vi "configuration UI.vi"() -> ()   [LabVIEW 2013, in "Scan Engine editor node.lvclass"]
uses:
  Scan Engine editor node.lvclass
  <vilib>/NI/Configuration Framework/Node/NodeRef.ctl
  <vilib>/NI/Configuration Framework/Node/NISE_CEF_Node.lvclass
  <vilib>/NI/AMC/Message Queue.ctl
  <vilib>/NI/AMC/Message.ctl
  <vilib>/NI/Tools/Keyed Array/KeyedArray.ctl
  <vilib>/NI/Configuration Framework/Node/UserEventRef.ctl
  <vilib>/NI/Configuration Framework/Controls/EventCluster.ctl
  module/configuration/Scan Engine configuration.lvclass
  <vilib>/Utility/miscctls.llb/LVComboBoxStrsAndValuesArrayTypeDef.ctl
  module/configuration/Scan Engine configuration.lvclass/Scan Engine configuration.ctl
  <vilib>/NI/Configuration Framework/serializable configuration/NISE_CEF_serializable configuration.lvclass/NISE_CEF_serializable configuration.ctl
  <vilib>/NI/Configuration Framework/serializable configuration/NISE_CEF_serializable configuration.lvclass
  Scan Engine editor node.lvclass/Scan Engine editor node.ctl
  <vilib>/NI/Tag Bus/tag/tag descriptor.lvclass/tag descriptor.ctl
  <vilib>/NI/Tag Bus Module Framework/module configuration/TBM module configuration.lvclass
  module/configuration/Write discover channels.vi
  module/configuration/Read discover channels.vi
  <vilib>/NI/Configuration Framework/serializable configuration/Read UID.vi
  <vilib>/NI/Tag Bus Data Framework/Configuration Editor/Classes/Module editor node/Read Module Configuration.vi
  read actual configuration.vi
  <vilib>/NI/Module Execution Interface/Engine Configuration/engine configuration.lvclass
  <vilib>/NI/Tag Bus Data Framework/Configuration Editor/Classes/Module editor node/module editor node.lvclass
  <vilib>/NI/Tag Bus/tag/tag descriptor.lvclass
  <vilib>/NI/Configuration Framework/NISE_CEF_TreeControl.lvlib
  <vilib>/NI/Tag Bus Data Framework/Configuration Editor/Classes/Engine Parent/Engine Parent Editor Node.lvclass
  <vilib>/Utility/miscctls.llb/LVRowAndColumnUnsignedTypeDef.ctl
  <vilib>/NI/Tools/Keyed Array/Tools_KeyedArray.lvlib
  <vilib>/NI/AMC/AMC.lvlib
panel:
  in  "hidden_settings":bool
  in  "Tab Control":enum32{"Static Configuration"}(tab)
  in  "Generate Tags":bool
  in  "Discover Channels?":bool
  in  "Remove Button":bool
  in  "Add Button":bool
  in  "channels":i32(listbox)
  in  "settings":bool
  in  "Import":bool
  in  "Tag":string(combo)
  in  "scan period (uSec)":u32=10000
  in  "user event":T1
  in  "main queue":T2
  in  "node ref":T3
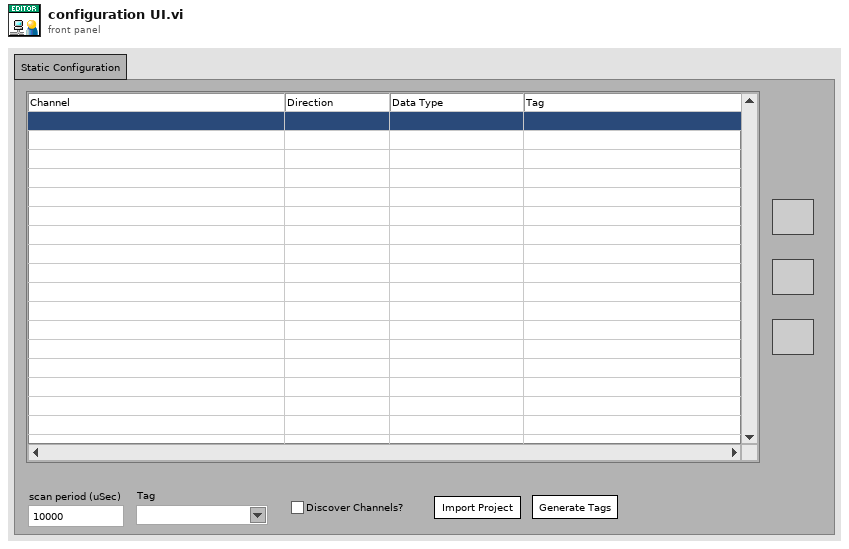
[diagram p1: front panel]
types:
  T1 = typedef "NISE_CEF_Node.lvclass/UserEventRef.ctl" = refnum<user-event>
  T2 = typedef "AMC.lvlib/Message Queue.ctl" = refnum<queue>
  T3 = typedef "NISE_CEF_Node.lvclass/NodeRef.ctl" = refnum<data-value>
  T4 = enum32{"invalid app kind", "Development System", "Run Time System", "Student Edition", "Embedded LabVIEW", "Evaluation", "Custom"}
  T5 = typedef "LVComboBoxStrsAndValuesArrayTypeDef.ctl" = cluster{"String":string, "Value":string}[]
  T6 = typedef "NISE_CEF_TreeControl.lvlib/EventCluster.ctl" = cluster{"command":string, "data":string}
  T7 = typedef "LVRowAndColumnUnsignedTypeDef.ctl" = cluster{"Row":u32, "Column":u32}
  T8 = typedef "Scan Engine editor node.lvclass/table line.ctl" = cluster{"tag":string, "channel":refnum<class "TBM channel.lvclass">}
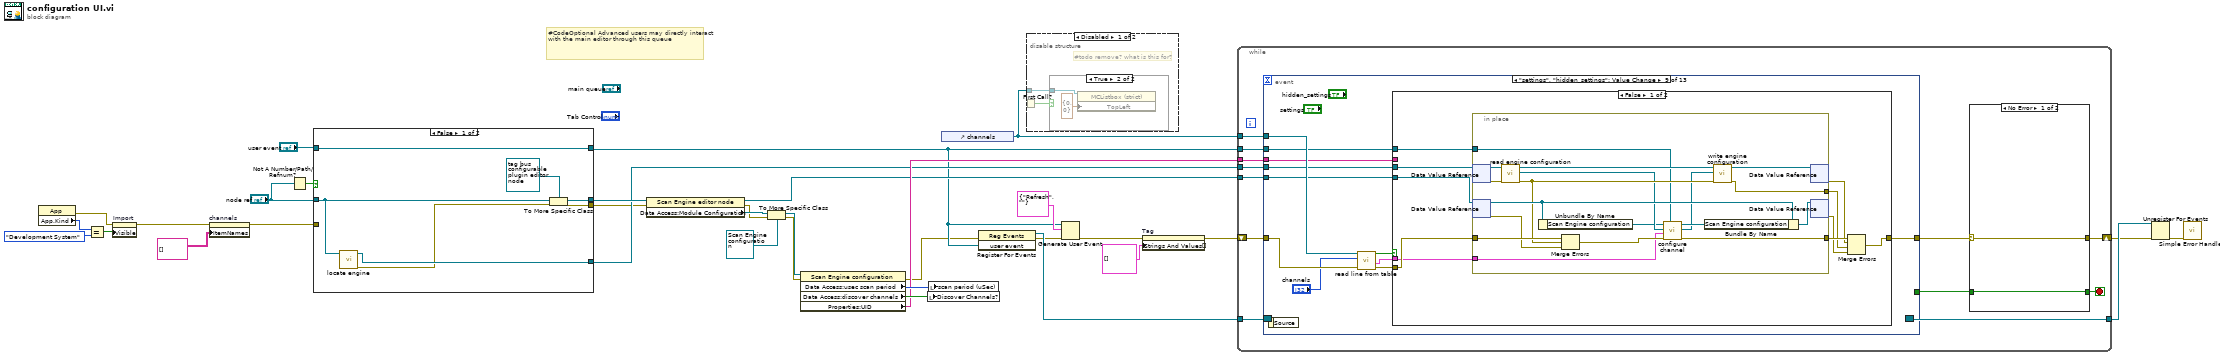
[diagram p0: block diagram]
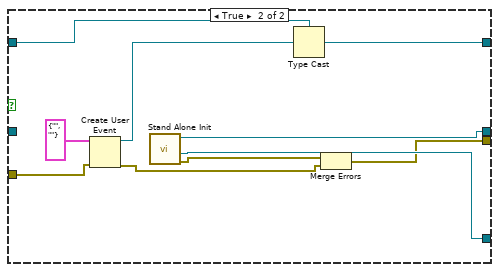
[diagram p4: hidden frame]
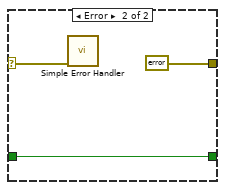
[diagram p5: hidden frame]
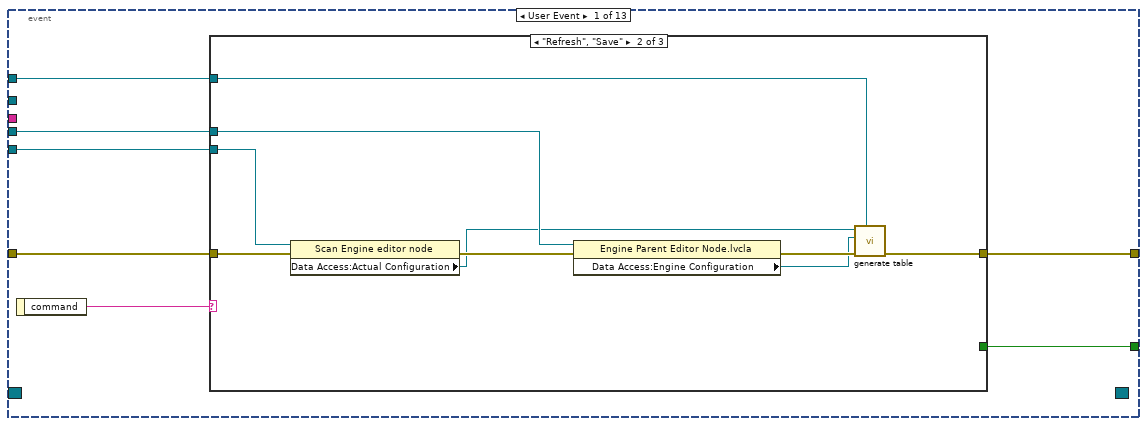
[diagram p6: hidden frame]
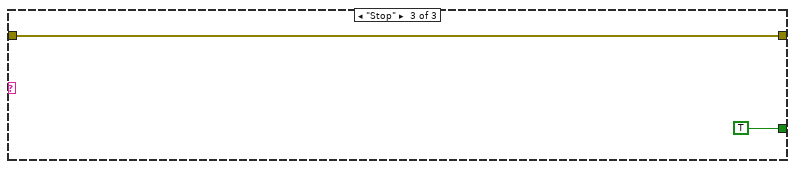
[diagram p8: hidden frame]
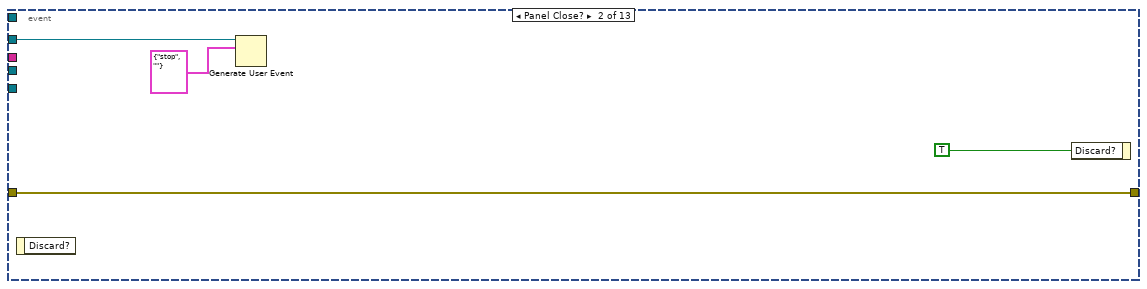
[diagram p9: hidden frame]
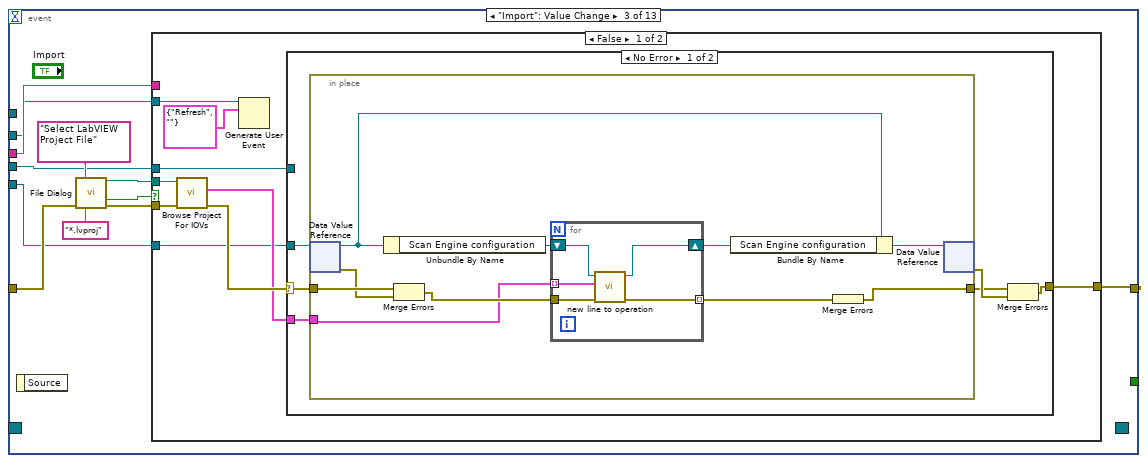
[diagram p10: hidden frame]
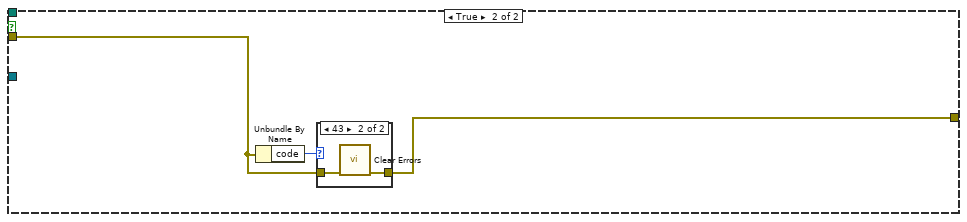
[diagram p12: hidden frame]
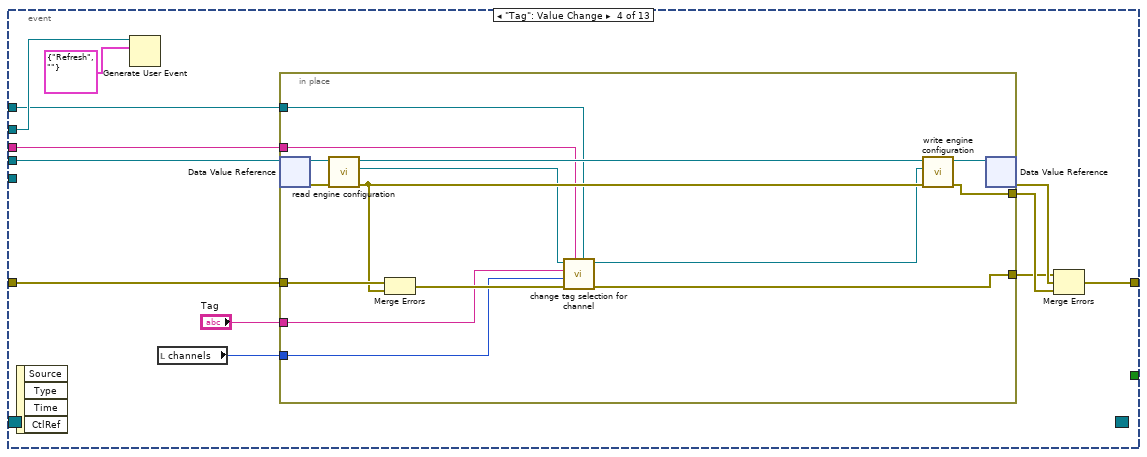
[diagram p14: hidden frame]
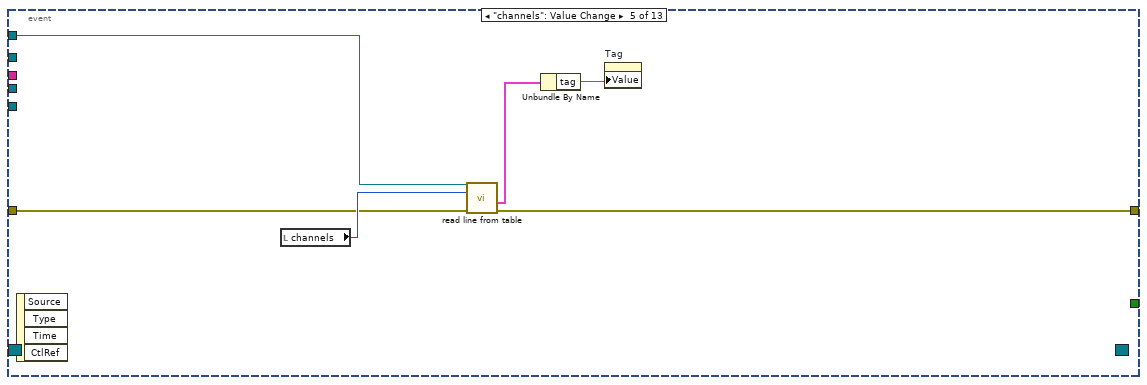
[diagram p15: hidden frame]
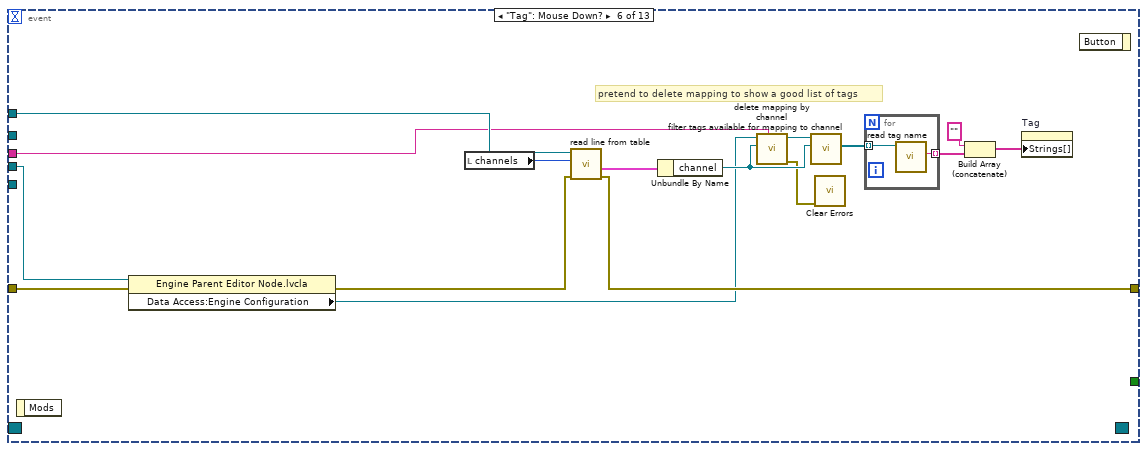
[diagram p16: hidden frame]
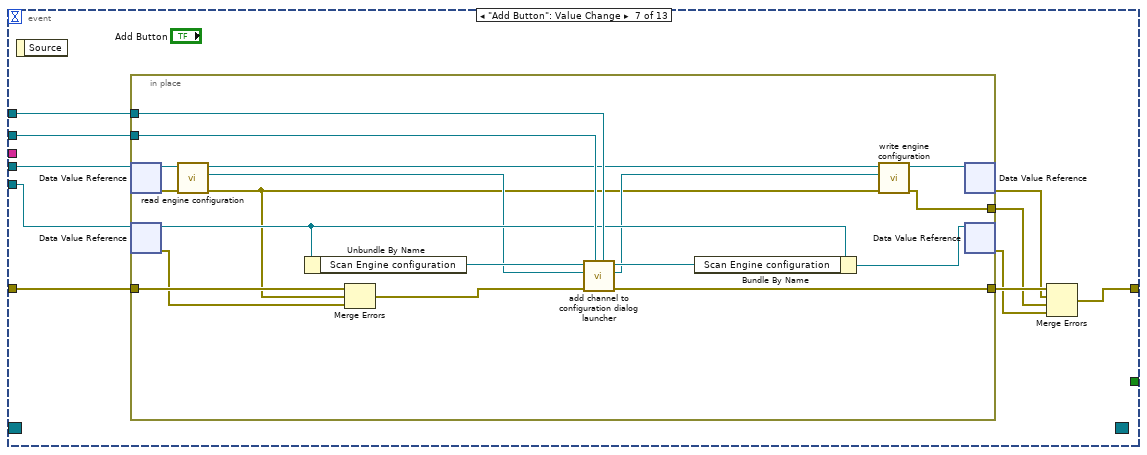
[diagram p17: hidden frame]
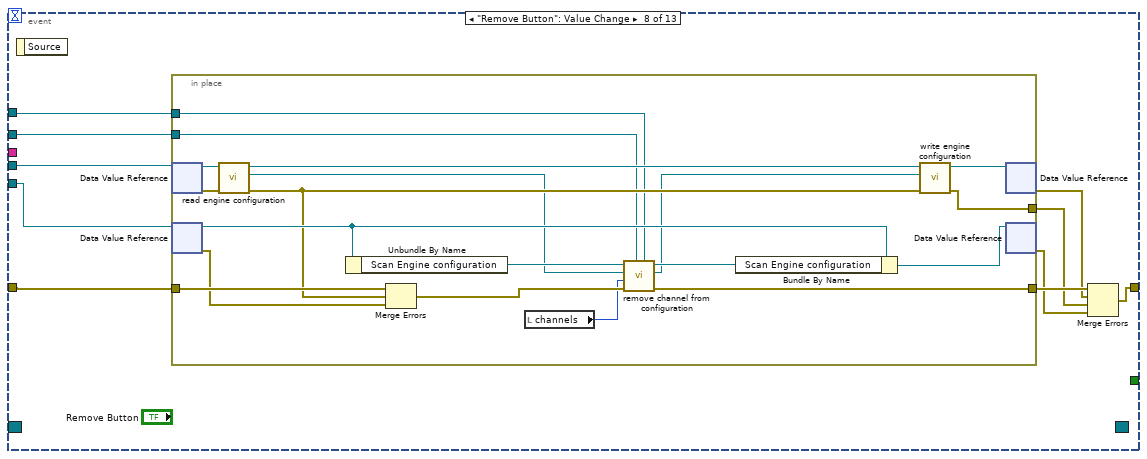
[diagram p18: hidden frame]
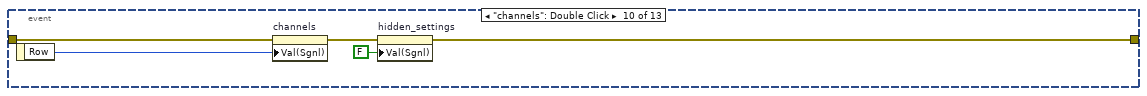
[diagram p20: hidden frame]
diagram:
  # "#CodeOptional Advanced users may directly interact with the main editor through this queue"
  n1 = property class="App"() -> (error out=w2:errorcluster, "App.Kind"=w5:T4)  [unwired: 2 in, 1 out]
  n2 = Equal?(x=w5, y=T4."Development System") -> (x = y?=w3:bool)
  n3 = property on="Import" class="Bool"(error in=w2, "Visible"=w3) -> (error out=w1:errorcluster)  [unwired: 1 in, 1 out]
  n4 = property on="channels" class="MCListbox (strict)"(error in=w1, "ItemNames"=string[][] [] ("Item Names")) -> (error out=w19:errorcluster)  [unwired: 1 in, 1 out]
  n5 = Not A Number/Path/Refnum?(number/path/refnum="node ref") -> (NaN/Path/Refnum?=w28:bool)
  n6 = case shown="False" w28 {
    tunnel: "user event" -> [w41 w42]
    tunnel: [w41 w43] -> w13
    tunnel: "node ref" -> [w39 _]
    tunnel: [w38 w51] -> w21
    tunnel: [w37 w45] -> w10
    tunnel: [w36 w49] -> w15
    tunnel: w19 -> [_ w46]
    frame False {
      n7 = call <vilib>:"locate engine.vi"("component"=w39) -> ("error out"=w35:errorcluster, "engine"=w36:refnum<data-value>)  [unwired: 9 in]
      n8 = To More Specific Class(target class=refnum<data-value> refnum ("data value reference"), reference=w39, error in=w35) -> (specific class reference=w38:refnum<data-value>, error out=w37:errorcluster)
    }
    frame True {
      n9 = Create User Event(user event datatype=T6 {"command"="", "data"=""} ("event data"), error in=w46) -> (user event=w47:refnum<user-event>, error out=w44:errorcluster)
      n10 = call "Stand Alone Init.vi"() -> ("error out"=w50:errorcluster, "Engine Parent Editor Node"=w49:refnum<data-value>, "Scan Engine Editor Node"=w51:refnum<data-value>)  [unwired: 9 in]
      n11 = Type Cast(type=w42, x=w47) -> (*(type *) &x=w43:T1)
      n12 = Merge Errors(w50, w44) -> (w45:errorcluster)
    }
  }
  n13 = property class="Scan Engine editor node"(reference=w21, error in=w10) -> (reference out=w16:refnum<data-value>, error out=w9:errorcluster, "Data Access:Module Configuration"=w24:refnum<class "TBM module configuration.lvclass">)
  n14 = To More Specific Class(target class=refnum<class "Scan Engine configuration.lvclass"> refnum ("Scan Engine configuration"), reference=w24, error in=w9) -> (specific class reference=w23:refnum<class "Scan Engine configuration.lvclass">, error out=w8:errorcluster)
  n15 = property class="Scan Engine configuration"(reference=w23, error in=w8) -> (error out=w7:errorcluster, "Data Access:usec scan period"=w30:u32, "Data Access:discover channels"=w29:bool, "Properties:UID"=w20:string)  [unwired: 1 out]
  n16 = local write "Discover Channels?"(w29) -> ()
  n17 = local write "scan period (uSec)"(w30) -> ()
  n18 = control-ref of="channels"() -> (w22:refnum<vi>)
  n19 = register-events(error in=w7, w13) -> (reference out=w34:refnum<event-registration>, error out=w12:errorcluster)  [unwired: 1 in]
  n20 = disable-structure shown="Disabled" {
    disable-tunnel: w22 -> [w52 _]
    frame Disabled {
      # "#todo remove? what is this for?"
      n21 = First Call?() -> (First Call?: T/F=w53:bool)
      n22 = case shown="True" w53 {
        tunnel: w52 -> [_ w54]
        frame False {
        }
        frame True {
          n23 = property class="MCListbox (strict)"(reference=w54, "TopLeft"=T7 {"Row"=0, "Column"=0} ("Top Left Visible Cell")) -> ()  [unwired: 1 in, 2 out]
        }
      }
    }
    frame Enabled {
    }
  }
  n24 = Generate User Event(user event=w13, event data cluster=T6 {"command"="Refresh", "data"=""} ("event data"), error in=w12) -> (error out=w11:errorcluster)  [unwired: 1 in, 1 out]
  n25 = property on="Tag" class="CmbBox"(error in=w11, "Strings And Values[]"=T5 [] ("Strings And Values []")) -> (error out=w31:errorcluster)  [unwired: 1 in, 1 out]
  n26 = while {
    tunnel: w34 -> [w67]
    tunnel: [w66] -> w33
    shift-right: [w62] -> w32
    shift-left: w31 -> [w65]
    tunnel: w22 -> [w57]
    tunnel: w20 -> [w61]
    tunnel: w16 -> [w59]
    tunnel: w15 -> [w58]
    tunnel: w13 -> [w56]
    stop <- w64 stop-if-true
    n27 = event shown="[8] \"settings\", \"hidden_settings\": Value Change" {
      selector: w67 -> [_ _ _ _ _ _ _ _ _ _ _ _ _]
      dyn-events: [_ _ _ _ _ _ _ _ _ _ _ _ _] -> w66
      timeout: _ -> [_ _ _ _ _ _ _ _ _ _ _ _ _]
      tunnel: [w78 _ _ _ _ _ _ _ _ _ _ _ _] -> w63
      tunnel: [w76 w95 w102 w151 w174 w185 w198 w228 w259 w294 w301 w316 w334] -> w60
      tunnel: w65 -> [w77 w95 w106 w150 w175 w184 w203 w227 w262 w296 w299 w314 w339]
      tunnel: w57 -> [w73 _ _ w148 w173 w189 w201 w223 w258 _ _ _ _]
      tunnel: w61 -> [_ _ w99 w149 _ w181 _ _ w257 _ _ _ w337]
      tunnel: w59 -> [w75 _ w96 _ _ _ w199 w226 w252 _ w300 w315 w332]
      tunnel: w58 -> [w74 _ w97 w144 _ w178 w200 w225 w253 _ _ _ w329]
      tunnel: w56 -> [_ w93 w98 w154 _ _ w202 w224 w255 _ _ _ w335]
      event User Event {
        n28 = event-data() -> ("command"=w79:string)  [unwired: 1 in]
        n29 = case shown="\"Refresh\", \"Save\"" w79 {
          tunnel: [_ _ TRUE] -> w78
          tunnel: w77 -> [w80 w88 w90]
          tunnel: [w80 w87 w90] -> w76
          tunnel: w75 -> [_ w84 _]
          tunnel: w74 -> [_ w83 _]
          tunnel: w73 -> [_ w89 _]
          frame Default {
          }
          frame "Refresh", "Save" {
            n30 = property class="Scan Engine editor node"(reference=w84, error in=w88) -> (error out=w86:errorcluster, "Data Access:Actual Configuration"=w81:refnum<class "Scan Engine configuration.lvclass">)  [unwired: 1 out]
            n31 = property class="Engine Parent Editor Node.lvcla"(reference=w83, error in=w86) -> (error out=w85:errorcluster, "Data Access:Engine Configuration"=w82:refnum<class "engine configuration.lvclass">)  [unwired: 1 out]
            n32 = call "generate table.vi"("table"=w89, "error in"=w85, "engine configuration in"=w82, "Scan Engine configuration"=w81) -> ("error out"=w87:errorcluster)  [unwired: 7 in]
          }
          frame "Stop" {
          }
        }
      }
      event Panel Close? {
        n33 = event-data() -> ()  [unwired: 1 in, 1 out]
        n34 = Generate User Event(user event=w93, event data cluster=T6 {"command"="stop", "data"=""} ("event data")) -> ()  [unwired: 2 in, 2 out]
        n35 = event-data("Discard?"=TRUE) -> ()  [unwired: 1 in, 1 out]
      }
      event "Import": Value Change {
        n36 = event-data() -> ()  [unwired: 1 in, 1 out]
        n37 = call "File Dialog"("prompt"="Select LabVIEW Project File", "error in"=w106, "pattern (all files)"="*.lvproj") -> ("selected path"=w101:path, "cancelled"=w104:bool, "error out"=w103:errorcluster)  [unwired: 9 in, 1 out]
        n38 = case shown="False" w104 {
          tunnel: w103 -> [w114 w139]
          tunnel: [w111 w138] -> w102
          tunnel: w101 -> [w115 _]
          tunnel: w99 -> [_ _]
          tunnel: w98 -> [w112 _]
          tunnel: w97 -> [w108 _]
          tunnel: w96 -> [w107 _]
          frame False {
            n39 = call "Browse Project For IOVs.vi"("error in"=w114, "Path"=w115) -> ("error out"=w110:errorcluster, "Tags"=w109:T8[])  [unwired: 8 in]
            n40 = Generate User Event(user event=w112, event data cluster=T6 {"command"="Refresh", "data"=""} ("event data")) -> ()  [unwired: 2 in, 2 out]
            n41 = case shown="No Error" w110 {
              selector: w110 -> [w119 w137]
              tunnel: [w120 w137] -> w111
              tunnel: w109 -> [w118 _]
              tunnel: w108 -> [_ _]
              tunnel: w107 -> [w117 _]
              frame No Error {
                n42 = in-place {
                  in-place-border: w119 -> [w131]
                  in-place-border: w118 -> [w124]
                  in-place-border: [w122] -> w116
                  n43 = in-place-dvr #1(w117) -> (w129:refnum<class "Scan Engine editor node.lvclass">, w130:errorcluster)
                  n44 = Unbundle By Name(w129) -> ("Scan Engine configuration"=w127:refnum<class "Scan Engine configuration.lvclass">)
                  n45 = Merge Errors(w131, w130) -> (w125:errorcluster)
                  n46 = for {
                    shift-right: [w134] -> w126
                    shift-left: w127 -> [w135]
                    tunnel: w125 -> [w133]
                    tunnel: w124 -> [w132] mode=indexing
                    tunnel: [w136] -> w123 mode=indexing
                    n47 = call "new line to operation.vi"("error in"=w133, "new line item"=w132, "Actual Configuration"=w135) -> ("error out"=w136:errorcluster, "Scan Engine configuration out"=w134:refnum<class "Scan Engine configuration.lvclass">)  [unwired: 4 in, 3 out]
                  }
                  n48 = Bundle By Name(cluster=w129, "Scan Engine configuration"=w126) -> (w128:refnum<class "Scan Engine editor node.lvclass">)
                  n49 = Merge Errors(w123) -> (w122:errorcluster)
                  n50 = in-place-dvr #1(w128) -> (w121:errorcluster)  [unwired: 1 out]
                }
                n51 = Merge Errors(w116, w121) -> (w120:errorcluster)
              }
              frame Error {
              }
            }
          }
          frame True {
            n52 = Unbundle By Name(w139) -> ("code"=w140:i32)
            n53 = case shown="43" w140 {
              tunnel: w139 -> [w141 w143]
              tunnel: [w141 w142] -> w138
              frame Default {
              }
              frame 43 {
                n54 = call <vilib>:"Clear Errors.vi"("error in (no error)"=w143) -> ("error out"=w142:errorcluster)  [unwired: 6 in]
              }
            }
          }
        }
      }
      event "Tag": Value Change {
        n55 = event-data() -> ()  [unwired: 1 in, 4 out]
        n56 = Generate User Event(user event=w154, event data cluster=T6 {"command"="Refresh", "data"=""} ("event data")) -> ()  [unwired: 2 in, 2 out]
        n57 = local read "channels"() -> (w145:i32)
        n58 = in-place {
          in-place-border: w149 -> [w158]
          in-place-border: w150 -> [w170]
          in-place-border: [w164] -> w153
          in-place-border: w148 -> [w162]
          in-place-border: [w161] -> w147
          in-place-border: "Tag" -> [w157]
          in-place-border: w145 -> [w156]
          n59 = in-place-dvr #2(w144) -> (w169:refnum<class "Engine Parent Editor Node.lvclass">, w168:errorcluster)
          n60 = call <vilib>:"read engine configuration.vi"("error in"=w168, "Engine Parent Editor Node in"=w169) -> ("error out"=w165:errorcluster, "engine configuration"=w159:refnum<class "engine configuration.lvclass">, "Engine Parent Editor Node out"=w167:refnum<class "Engine Parent Editor Node.lvclass">)  [unwired: 7 in]
          n61 = Merge Errors(w170, w165) -> (w163:errorcluster)
          n62 = call "change tag selection for channel.vi"("channels table"=w162, "instance identifier"=w158, "error in"=w163, "channels"=w156, "Tag"=w157, "engine configuration in"=w159) -> ("error out"=w161:errorcluster, "engine configuration out"=w160:refnum<class "engine configuration.lvclass">)  [unwired: 4 in]
          n63 = call <vilib>:"write engine configuration.vi"("error in"=w165, "engine configuration"=w160, "Engine Parent Editor Node in"=w167) -> ("error out"=w164:errorcluster, "Engine Parent Editor Node out"=w166:refnum<class "Engine Parent Editor Node.lvclass">)  [unwired: 7 in]
          n64 = in-place-dvr #2(w166) -> (w152:errorcluster)  [unwired: 1 out]
        }
        n65 = Merge Errors(w147, w152, w153) -> (w151:errorcluster)
      }
      event "channels": Value Change {
        n66 = event-data() -> ()  [unwired: 1 in, 4 out]
        n67 = local read "channels"() -> (w176:i32)
        n68 = call "read line from table.vi"("error in"=w175, "line number"=w176, "operations table"=w173) -> ("error out"=w174:errorcluster, "line"=w172:T8)  [unwired: 5 in, 2 out]
        n69 = Unbundle By Name(w172) -> ("tag"=w171:string)
        n70 = property on="Tag" class="CmbBox"("Value"=w171) -> ()  [unwired: 2 in, 2 out]
      }
      event "Tag": Mouse Down? {
        # "pretend to delete mapping to show a good list of tags"
        n71 = event-data() -> ()  [unwired: 1 in, 1 out]
        n72 = property class="Engine Parent Editor Node.lvcla"(reference=w178, error in=w184) -> (error out=w179:errorcluster, "Data Access:Engine Configuration"=w177:refnum<class "engine configuration.lvclass">)  [unwired: 1 out]
        n73 = local read "channels"() -> (w188:i32)
        n74 = call "read line from table.vi"("error in"=w179, "line number"=w188, "operations table"=w189) -> ("error out"=w185:errorcluster, "line"=w187:T8)  [unwired: 5 in, 2 out]
        n75 = Unbundle By Name(w187) -> ("channel"=w182:refnum<class "TBM channel.lvclass">)
        n76 = call <vilib>:"delete mapping by channel.vi"("owner ID"=w181, "channel"=w182, "engine configuration in"=w177) -> ("error out"=w180:errorcluster, "engine configuration out"=w183:refnum<class "engine configuration.lvclass">)  [unwired: 7 in]
        n77 = call <vilib>:"filter tags available for mapping to channel.vi"("channel to map to"=w182, "engine configuration in"=w183) -> ("filtered tags"=w192:refnum<class "tag descriptor.lvclass">[])  [unwired: 8 in, 1 out]
        n78 = call <vilib>:"Clear Errors.vi"("error in (no error)"=w180) -> ()  [unwired: 6 in, 1 out]
        n79 = for {
          tunnel: w192 -> [w194] mode=indexing
          tunnel: [w193] -> w191 mode=indexing
          n80 = call <vilib>:"read tag name.vi"("system tag in"=w194) -> ("name"=w193:string)  [unwired: 8 in, 2 out]
        }
        n81 = Build Array (concatenate)("", w191) -> (w186:string[])
        n82 = property on="Tag" class="CmbBox"("Strings[]"=w186) -> ()  [unwired: 2 in, 2 out]
        n83 = event-data() -> ()  [unwired: 2 in, 1 out]
      }
      event "Add Button": Value Change {
        n84 = event-data() -> ()  [unwired: 1 in, 1 out]
        n85 = in-place {
          in-place-border: [w222] -> w204
          in-place-border: w203 -> [w221]
          in-place-border: w202 -> [w220]
          in-place-border: w201 -> [w219]
          in-place-border: [w210] -> w196
          n86 = in-place-dvr #3(w200) -> (w217:refnum<class "Engine Parent Editor Node.lvclass">, w216:errorcluster)
          n87 = in-place-dvr #4(w199) -> (w213:refnum<class "Scan Engine editor node.lvclass">, w215:errorcluster)
          n88 = call <vilib>:"read engine configuration.vi"("error in"=w216, "Engine Parent Editor Node in"=w217) -> ("error out"=w205:errorcluster, "engine configuration"=w207:refnum<class "engine configuration.lvclass">, "Engine Parent Editor Node out"=w208:refnum<class "Engine Parent Editor Node.lvclass">)  [unwired: 7 in]
          n89 = Unbundle By Name(w213) -> ("Scan Engine configuration"=w214:refnum<class "Scan Engine configuration.lvclass">)
          n90 = Merge Errors(w221, w205, w215) -> (w218:errorcluster)
          n91 = call "add channel to configuration dialog launcher.vi"("channels"=w219, "user event"=w220, "error in"=w218, "engine configuration.lvclass in"=w207, "Scan Engine configuration in"=w214) -> ("error out"=w222:errorcluster, "engine configuration.lvclass out"=w206:refnum<class "engine configuration.lvclass">, "Scan Engine configuration out"=w212:refnum<class "Scan Engine configuration.lvclass">)  [unwired: 4 in]
          n92 = Bundle By Name(cluster=w213, "Scan Engine configuration"=w212) -> (w211:refnum<class "Scan Engine editor node.lvclass">)
          n93 = call <vilib>:"write engine configuration.vi"("error in"=w205, "engine configuration"=w206, "Engine Parent Editor Node in"=w208) -> ("error out"=w210:errorcluster, "Engine Parent Editor Node out"=w209:refnum<class "Engine Parent Editor Node.lvclass">)  [unwired: 7 in]
          n94 = in-place-dvr #3(w209) -> (w195:errorcluster)  [unwired: 1 out]
          n95 = in-place-dvr #4(w211) -> (w197:errorcluster)  [unwired: 1 out]
        }
        n96 = Merge Errors(w204, w195, w196, w197) -> (w198:errorcluster)
      }
      event "Remove Button": Value Change {
        n97 = event-data() -> ()  [unwired: 1 in, 1 out]
        n98 = in-place {
          in-place-border: [w239] -> w232
          in-place-border: w227 -> [w251]
          in-place-border: w224 -> [w240]
          in-place-border: w223 -> [w241]
          in-place-border: [w245] -> w230
          n99 = in-place-dvr #5(w225) -> (w250:refnum<class "Engine Parent Editor Node.lvclass">, w249:errorcluster)
          n100 = in-place-dvr #6(w226) -> (w247:refnum<class "Scan Engine editor node.lvclass">, w248:errorcluster)
          n101 = call <vilib>:"read engine configuration.vi"("error in"=w249, "Engine Parent Editor Node in"=w250) -> ("error out"=w242:errorcluster, "engine configuration"=w234:refnum<class "engine configuration.lvclass">, "Engine Parent Editor Node out"=w243:refnum<class "Engine Parent Editor Node.lvclass">)  [unwired: 7 in]
          n102 = Unbundle By Name(w247) -> ("Scan Engine configuration"=w237:refnum<class "Scan Engine configuration.lvclass">)
          n103 = Merge Errors(w251, w242, w248) -> (w238:errorcluster)
          n104 = local read "channels"() -> (w233:i32)
          n105 = call "remove channel from configuration.vi"("channels"=w241, "user event"=w240, "error in"=w238, "channels value"=w233, "engine configuration in"=w234, "Scan Engine configuration in"=w237) -> ("error out"=w239:errorcluster, "engine configuration out"=w235:refnum<class "engine configuration.lvclass">, "Scan Engine configuration out"=w236:refnum<class "Scan Engine configuration.lvclass">)  [unwired: 3 in]
          n106 = Bundle By Name(cluster=w247, "Scan Engine configuration"=w236) -> (w246:refnum<class "Scan Engine editor node.lvclass">)
          n107 = call <vilib>:"write engine configuration.vi"("error in"=w242, "engine configuration"=w235, "Engine Parent Editor Node in"=w243) -> ("error out"=w245:errorcluster, "Engine Parent Editor Node out"=w244:refnum<class "Engine Parent Editor Node.lvclass">)  [unwired: 7 in]
          n108 = in-place-dvr #5(w244) -> (w229:errorcluster)  [unwired: 1 out]
          n109 = in-place-dvr #6(w246) -> (w231:errorcluster)  [unwired: 1 out]
        }
        n110 = Merge Errors(w232, w229, w230, w231) -> (w228:errorcluster)
      }
      event "settings", "hidden_settings": Value Change {
        n111 = event-data() -> ()  [unwired: 1 in, 1 out]
        n112 = call "read line from table.vi"("error in"=w262, "line number"="channels", "operations table"=w258) -> ("error out"=w261:errorcluster, "line"=w256:T8, "empty channel?"=w254:bool)  [unwired: 5 in, 1 out]
        n113 = case shown="False" w254 {
          tunnel: w261 -> [w265 w291]
          tunnel: [w268 w291] -> w259
          tunnel: w257 -> [_ _]
          tunnel: w256 -> [w264 _]
          tunnel: w255 -> [w263 _]
          tunnel: w253 -> [w267 _]
          tunnel: w252 -> [w266 _]
          frame False {
            n114 = in-place {
              in-place-border: [w279] -> w272
              in-place-border: w265 -> [w290]
              in-place-border: w263 -> [w273]
              in-place-border: [w284] -> w270
              in-place-border: w264 -> [w274]
              n115 = in-place-dvr #7(w267) -> (w289:refnum<class "Engine Parent Editor Node.lvclass">, w288:errorcluster)
              n116 = in-place-dvr #8(w266) -> (w286:refnum<class "Scan Engine editor node.lvclass">, w287:errorcluster)
              n117 = call <vilib>:"read engine configuration.vi"("error in"=w288, "Engine Parent Editor Node in"=w289) -> ("error out"=w281:errorcluster, "engine configuration"=w276:refnum<class "engine configuration.lvclass">, "Engine Parent Editor Node out"=w282:refnum<class "Engine Parent Editor Node.lvclass">)  [unwired: 7 in]
              n118 = Unbundle By Name(w286) -> ("Scan Engine configuration"=w275:refnum<class "Scan Engine configuration.lvclass">)
              n119 = Merge Errors(w290, w281, w287) -> (w280:errorcluster)
              n120 = call "configure channel.vi"("user event"=w273, "error in"=w280, "line"=w274, "engine configuration in"=w276, "Scan Engine configuration in"=w275) -> ("error out"=w279:errorcluster, "engine configuration out"=w277:refnum<class "engine configuration.lvclass">, "Scan Engine configuration out"=w278:refnum<class "Scan Engine configuration.lvclass">)  [unwired: 4 in]
              n121 = Bundle By Name(cluster=w286, "Scan Engine configuration"=w278) -> (w285:refnum<class "Scan Engine editor node.lvclass">)
              n122 = call <vilib>:"write engine configuration.vi"("error in"=w281, "engine configuration"=w277, "Engine Parent Editor Node in"=w282) -> ("error out"=w284:errorcluster, "Engine Parent Editor Node out"=w283:refnum<class "Engine Parent Editor Node.lvclass">)  [unwired: 7 in]
              n123 = in-place-dvr #7(w283) -> (w269:errorcluster)  [unwired: 1 out]
              n124 = in-place-dvr #8(w285) -> (w271:errorcluster)  [unwired: 1 out]
            }
            n125 = Merge Errors(w272, w269, w270, w271) -> (w268:errorcluster)
          }
          frame True {
          }
        }
      }
      event "channels": Double Click {
        n126 = event-data() -> ("Row"=w292:i32)  [unwired: 1 in]
        n127 = property on="channels" class="MCListbox (strict)"(error in=w296, "Val(Sgnl)"=w292) -> (error out=w295:errorcluster)  [unwired: 1 in, 1 out]
        n128 = property on="hidden_settings" class="Bool (strict)"(error in=w295, "Val(Sgnl)"=FALSE ("Value (Signaling)")) -> (error out=w294:errorcluster)  [unwired: 1 in, 1 out]
      }
      event "scan period (uSec)": Value Change {
        n129 = event-data() -> ()  [unwired: 1 in, 1 out]
        n130 = in-place {
          in-place-border: w299 -> [w311]
          in-place-border: [w304] -> w298
          in-place-border: "scan period (uSec)" -> [w303]
          n131 = in-place-dvr #9(w300) -> (w309:refnum<class "Scan Engine editor node.lvclass">, w310:errorcluster)
          n132 = Unbundle By Name(w309) -> ("Scan Engine configuration"=w306:refnum<class "Scan Engine configuration.lvclass">)
          n133 = Merge Errors(w311, w310) -> (w307:errorcluster)
          n134 = property class="Scan Engine configuration"(reference=w306, error in=w307, "Data Access:usec scan period"=w303) -> (reference out=w305:refnum<class "Scan Engine configuration.lvclass">, error out=w304:errorcluster)
          n135 = Bundle By Name(cluster=w309, "Scan Engine configuration"=w305) -> (w308:refnum<class "Scan Engine editor node.lvclass">)
          n136 = in-place-dvr #9(w308) -> (w302:errorcluster)  [unwired: 1 out]
        }
        n137 = Merge Errors(w298, w302) -> (w301:errorcluster)
      }
      event "Discover Channels?": Value Change {
        n138 = event-data() -> ()  [unwired: 1 in, 3 out]
        n139 = in-place {
          in-place-border: w314 -> [w326]
          in-place-border: [w319] -> w313
          in-place-border: "Discover Channels?" -> [w318]
          n140 = in-place-dvr #10(w315) -> (w324:refnum<class "Scan Engine editor node.lvclass">, w325:errorcluster)
          n141 = Unbundle By Name(w324) -> ("Scan Engine configuration"=w321:refnum<class "Scan Engine configuration.lvclass">)
          n142 = Merge Errors(w326, w325) -> (w322:errorcluster)
          n143 = property class="Scan Engine configuration"(reference=w321, error in=w322, "Data Access:discover channels"=w318) -> (reference out=w320:refnum<class "Scan Engine configuration.lvclass">, error out=w319:errorcluster)
          n144 = Bundle By Name(cluster=w324, "Scan Engine configuration"=w320) -> (w323:refnum<class "Scan Engine editor node.lvclass">)
          n145 = in-place-dvr #10(w323) -> (w317:errorcluster)  [unwired: 1 out]
        }
        n146 = Merge Errors(w313, w317) -> (w316:errorcluster)
      }
      event "Generate Tags": Value Change {
        # "#todo Create an engine filter VI that returns all channels that are currently mapped."
        n147 = event-data() -> ()  [unwired: 1 in, 1 out]
        n148 = property class="Scan Engine editor node"(reference=w332, error in=w339) -> (error out=w333:errorcluster, "Data Access:Module Configuration"=w331:refnum<class "TBM module configuration.lvclass">)  [unwired: 1 out]
        n149 = Generate User Event(user event=w335, event data cluster=T6 {"command"="Refresh", "data"=""} ("event data")) -> ()  [unwired: 2 in, 2 out]
        n150 = call-dynamic "get channels.vi"("module configuration in"=w331) -> ("channels"=w330:refnum<class "TBM channel.lvclass">[])  [unwired: 9 in, 1 out]
        n151 = in-place {
          in-place-border: [w352] -> w338
          in-place-border: w337 -> [w351]
          in-place-border: w333 -> [w350]
          in-place-border: w330 -> [w349]
          in-place-border: [w340] -> w328
          n152 = in-place-dvr #11(w329) -> (w348:refnum<class "Engine Parent Editor Node.lvclass">, w347:errorcluster)
          n153 = call <vilib>:"read engine configuration.vi"("error in"=w347, "Engine Parent Editor Node in"=w348) -> ("error out"=w342:errorcluster, "engine configuration"=w343:refnum<class "engine configuration.lvclass">, "Engine Parent Editor Node out"=w346:refnum<class "Engine Parent Editor Node.lvclass">)  [unwired: 7 in]
          n154 = Merge Errors(w350, w342) -> (w341:errorcluster)
          n155 = case shown="No Error" w341 {
            selector: w341 -> [w353 w380]
            tunnel: [w358 w379] -> w352
            tunnel: w351 -> [w357 _]
            tunnel: w349 -> [w356 _]
            tunnel: [w355 w381] -> w344
            tunnel: w343 -> [w354 w381]
            frame No Error {
              n156 = for {
                tunnel: w356 -> [w359] mode=indexing
                shift-right: [w367] -> w355
                shift-left: w354 -> [w365]
                tunnel: w357 -> [w364]
                tunnel: w353 -> [w361]
                tunnel: [w366] -> w358 mode=indexing
                n157 = call "simplify scan engine channel name.vi"("scan engine channel in"=w359) -> ("simplified channel"=w360:refnum<class "TBM channel.lvclass">)  [unwired: 10 in]
                n158 = call <vilib>:"find tag mapped to channel.vi"("owner"=w364, "error in"=w361, "channel"=w360, "engine configuration in"=w365) -> ("error out"=w362:errorcluster, "engine configuration out"=w363:refnum<class "engine configuration.lvclass">)  [unwired: 5 in, 1 out]
                n159 = case shown="Error" w362 {
                  selector: w362 -> [w368 _]
                  tunnel: [w369 w376] -> w367
                  tunnel: [w368 w375] -> w366
                  tunnel: w364 -> [_ w374]
                  tunnel: w360 -> [_ w373]
                  tunnel: w363 -> [w369 w372]
                  tunnel: w361 -> [_ w371]
                  tunnel: w359 -> [_ w370]
                  frame No Error {
                  }
                  frame Error {
                    n160 = call <vilib>:"add tag.vi"("error in"=w371, "tag descriptor"=w373, "engine configuration in"=w372) -> ("error out"=w377:errorcluster, "engine configuration out"=w378:refnum<class "engine configuration.lvclass">)  [unwired: 7 in]
                    n161 = call <vilib>:"add mapping.vi"("owner ID"=w374, "error in"=w377, "channel"=w370, "tag descriptor"=w373, "engine configuration"=w378) -> ("error out"=w375:errorcluster, "engine configuration out"=w376:refnum<class "engine configuration.lvclass">)  [unwired: 5 in]
                  }
                }
              }
            }
            frame Error {
              n162 = Build Array(w380) -> (w379:errorcluster[])
            }
          }
          n163 = call <vilib>:"write engine configuration.vi"("error in"=w342, "engine configuration"=w344, "Engine Parent Editor Node in"=w346) -> ("error out"=w340:errorcluster, "Engine Parent Editor Node out"=w345:refnum<class "Engine Parent Editor Node.lvclass">)  [unwired: 7 in]
          n164 = in-place-dvr #11(w345) -> (w327:errorcluster)  [unwired: 1 out]
        }
        n165 = Merge Errors(w327, w328, w338) -> (w334:errorcluster)
      }
    }
    n166 = case shown="No Error" w60 {
      selector: w60 -> [w68 w71]
      tunnel: [w69 w72] -> w64
      tunnel: w63 -> [w69 w72]
      tunnel: [w68 errorcluster {"status"=FALSE, "code"=0, "source"=""} ("error out")] -> w62
      frame No Error {
      }
      frame Error {
        n167 = call <vilib>:"Simple Error Handler.vi"("error in (no error)"=w71) -> ()  [unwired: 4 in, 5 out]
      }
    }
  }
  n168 = Unregister For Events(event registration refnum=w33, error in=w32) -> (error out=w17:errorcluster)
  n169 = call <vilib>:"Simple Error Handler.vi"("error in (no error)"=w17) -> ()  [unwired: 4 in, 5 out]
